vi "Calculator___Casestructer.vi"() -> ()   [LabVIEW 2019]
doc: "Calculator_1\nBy Mohammad Sabouri\nmohamadsabora@yahoo.com"
panel:
  in  "Radio Buttons":T1(radio)
  out "Output":dbl
  in  "Num2":dbl
  in  "Num1":dbl
  in  "stop":bool
  # "Calculator_1\nBy Mohammad Sabouri\nmohammadsabory@yahoo.com"
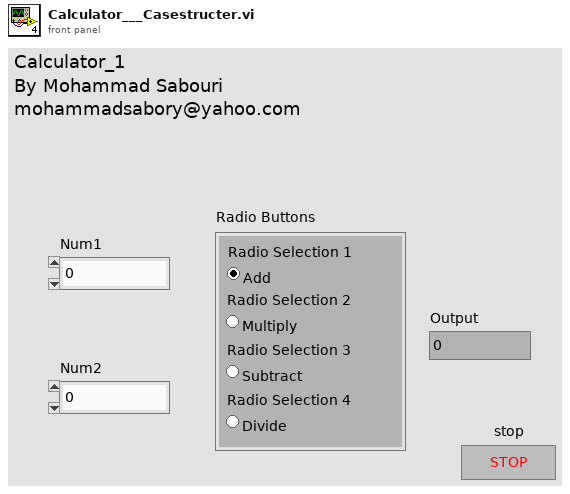
[diagram p1: front panel]
types:
  T1 = enum32{"Radio Selection 1", "Radio Selection 2", "Radio Selection 3", "Radio Selection 4"}
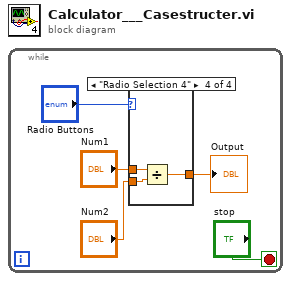
[diagram p0: block diagram]
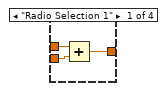
[diagram p2: hidden frame]
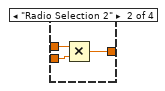
[diagram p3: hidden frame]
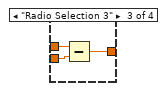
[diagram p4: hidden frame]
diagram:
  n1 = while {
    stop <- "stop" stop-if-true
    n2 = case shown="\"Radio Selection 4\"" "Radio Buttons" {
      tunnel: "Num1" -> [w8 w11 w14 w17]
      tunnel: "Num2" -> [w7 w10 w13 w16]
      tunnel: [w6 w9 w12 w15] -> w1
      frame "Radio Selection 1" {
        n3 = Add(x=w8, y=w7) -> (x+y=w6:dbl)
      }
      frame "Radio Selection 2" {
        n4 = Multiply(x=w11, y=w10) -> (x*y=w9:dbl)
      }
      frame "Radio Selection 3" {
        n5 = Subtract(x=w14, y=w13) -> (x-y=w12:dbl)
      }
      frame "Radio Selection 4" {
        n6 = Divide(x=w17, y=w16) -> (x/y=w15:dbl)
      }
    }
    "Output" <- w1
  }
